vi "Close XWPF Writer.vi"(8 "error in (no error)":errorcluster, 11 "xwpfWriter in":refnum<class "xwpfWriter.lvclass">) -> (0 "error out":errorcluster, 3 "xwpfWriter out":refnum<class "xwpfWriter.lvclass">)   [LabVIEW 2017, in "LabVIEW NPOI.lvlib" / "xwpfWriter.lvclass"]
doc: "Closes the XWPFDocument and the XWPFExtractor references."
uses:
  xwpfWriter.lvclass
  xwpfWriter.lvclass/xwpfWriter.ctl
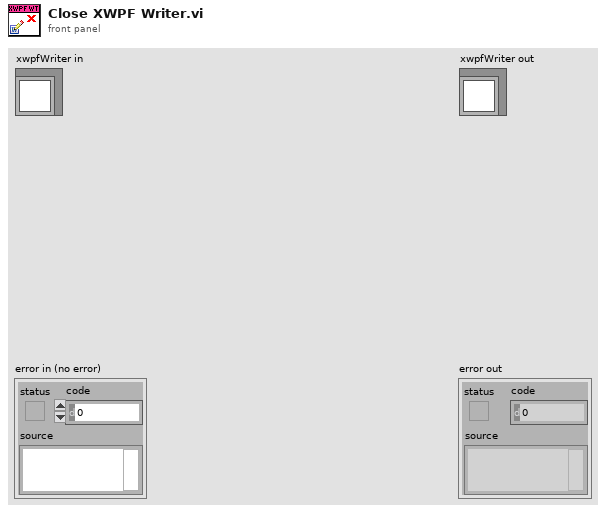
[diagram p1: front panel]
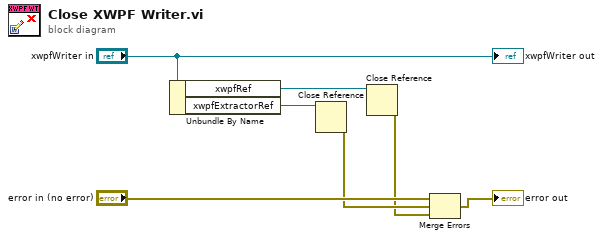
[diagram p0: block diagram]
diagram:
  n1 = Unbundle By Name("xwpfWriter in") -> ("xwpfRef"=w2:refnum<k24>, "xwpfExtractorRef"=w4:refnum<k24>)
  n2 = Close Reference(reference=w4) -> (error out=w3:errorcluster)  [unwired: 1 in]
  n3 = Close Reference(reference=w2) -> (error out=w1:errorcluster)  [unwired: 1 in]
  n4 = Merge Errors("error in (no error)", w3, w1) -> (→"error out":errorcluster)
  "xwpfWriter out" <- "xwpfWriter in"
